vi "niRFUtil MT UTIL Generate Fractional Resampler FIR Coefficients v2.vi"() -> (0 "effective filter length":i32, 1 "interpolation factor":i32, 2 "extended length":i32, 3 "polyphase filter":T1 min=0 max=127 format="%.2f")   [LabVIEW 2015, in "niRFUtil.lvlib"]
uses:
  niRFUtil.lvlib
  Includes/niRFUtil INC Real Array.ctl
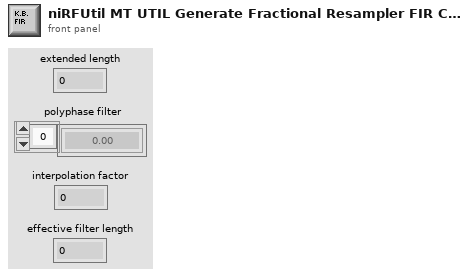
[diagram p1: front panel]
types:
  T1 = typedef "niRFUtil.lvlib/niRFUtil INC Real Array.ctl" = sgl[]
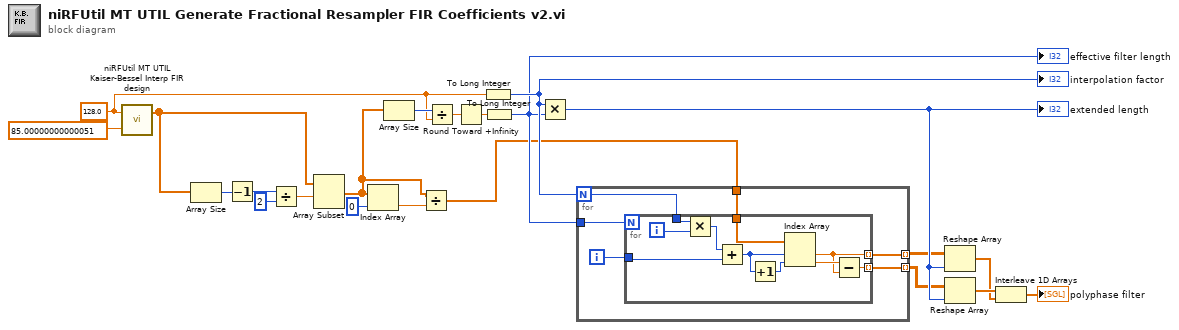
[diagram p0: block diagram]
diagram:
  w3 = 128.0 ("interpolation factor")
  n1 = call "niRFUtil MT UTIL Kaiser-Bessel Interp FIR design.vi"("Stop Attenuation"=85.00000000000051, "interpolation factor"=w3) -> ("h"=w1:T1)  [unwired: 1 in]
  n2 = Array Size(array=w1) -> (size(s)=w17:i32)
  n3 = Decrement(x=w17) -> (x-1=w16:i32)
  n4 = Divide(x=w16, y=2) -> (x/y=w14:dbl)
  n5 = Array Subset(array=w1, index=w14) -> (w5:T1)  [unwired: 1 in]
  n6 = Index Array(array=w5, index=0) -> (element=w6:sgl)
  n7 = Array Size(array=w5) -> (size(s)=w22:i32)
  n8 = Divide(x=w5, y=w6) -> (x/y=w4:T1)
  n9 = Divide(x=w22, y=w3) -> (x/y=w21:dbl)
  n10 = Round Toward +Infinity(x=w21) -> (ceil(x): smallest int >= x=w20:dbl)
  n11 = To Long Integer(number=w3) -> (32bit integer=w19:i32)
  "interpolation factor" <- w19
  n12 = To Long Integer(number=w20) -> (32bit integer=w18:i32)
  "effective filter length" <- w18
  n13 = Multiply(x=w19, y=w18) -> (x*y=w13:i32)
  "extended length" <- w13
  n14 = for {
    N: w19 -> [w27]
    tunnel: w4 -> [w26]
    tunnel: [w25] -> w12 mode=indexing
    tunnel: w18 -> [w24]
    tunnel: [w23] -> w11 mode=indexing
    i -> [w28]
    n15 = for {
      N: w24 -> [_]
      tunnel: w28 -> [w35]
      tunnel: w27 -> [w37]
      tunnel: w26 -> [w34]
      tunnel: [w30] -> w25 mode=indexing
      tunnel: [w29] -> w23 mode=indexing
      i -> [w38]
      n16 = Multiply(x=w37, y=w38) -> (x*y=w36:i32)
      n17 = Add(x=w36, y=w35) -> (x+y=w32:i32)
      n18 = Increment(x=w32) -> (x+1=w33:i32)
      n19 = Index Array(array=w34, index #1=w32, index #2=w33) -> (element #1=w30:sgl, element #2=w31:sgl)
      n20 = Subtract(x=w31, y=w30) -> (x-y=w29:sgl)
    }
  }
  n21 = Reshape Array(w12, w13) -> (w9:sgl[])
  n22 = Reshape Array(w11, w13) -> (w10:sgl[])
  n23 = Interleave 1D Arrays(w10, w9) -> (→"polyphase filter":sgl[])
